vi "py_accel.vi"(7 "Time Target (s)":dbl=1.0, 8 "error in":errorcluster, 10 "Accel CSV file":path, 11 "COM":refnum<visa-resource-name>) -> (2 "File OK":bool, 3 "Com\nError":bool)   [LabVIEW 2021]
uses:
  <vilib>/Instr/_visa.llb/VISA Flush IO Buffer Mask.ctl
panel:
  out "read buffer":string
  # "acc,ms timer refernce,x_accel,y_accel,z_accel   [m/s^2]"
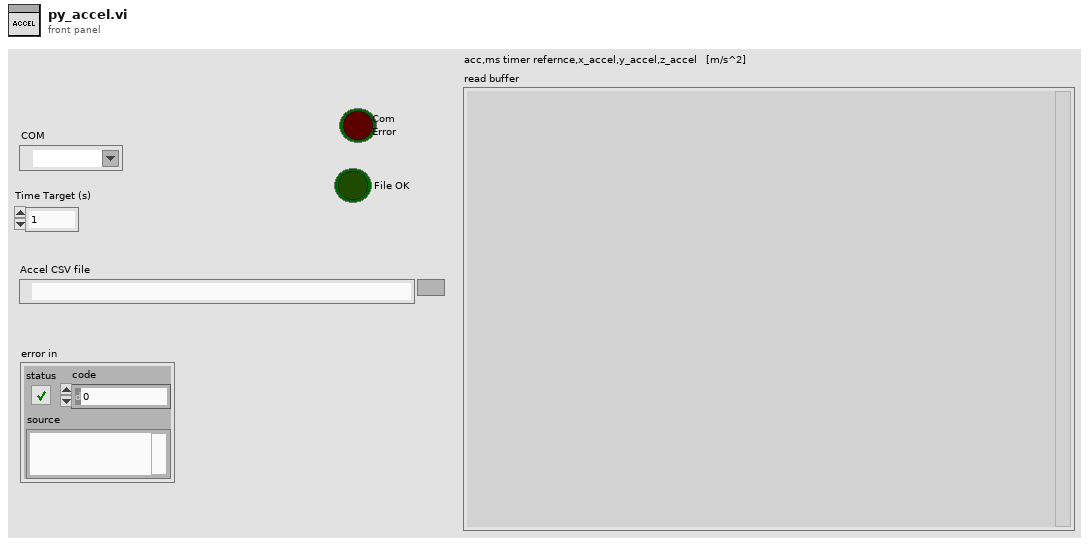
[diagram p1: front panel]
types:
  T1 = typedef "VISA Flush IO Buffer Mask.ctl" = u16
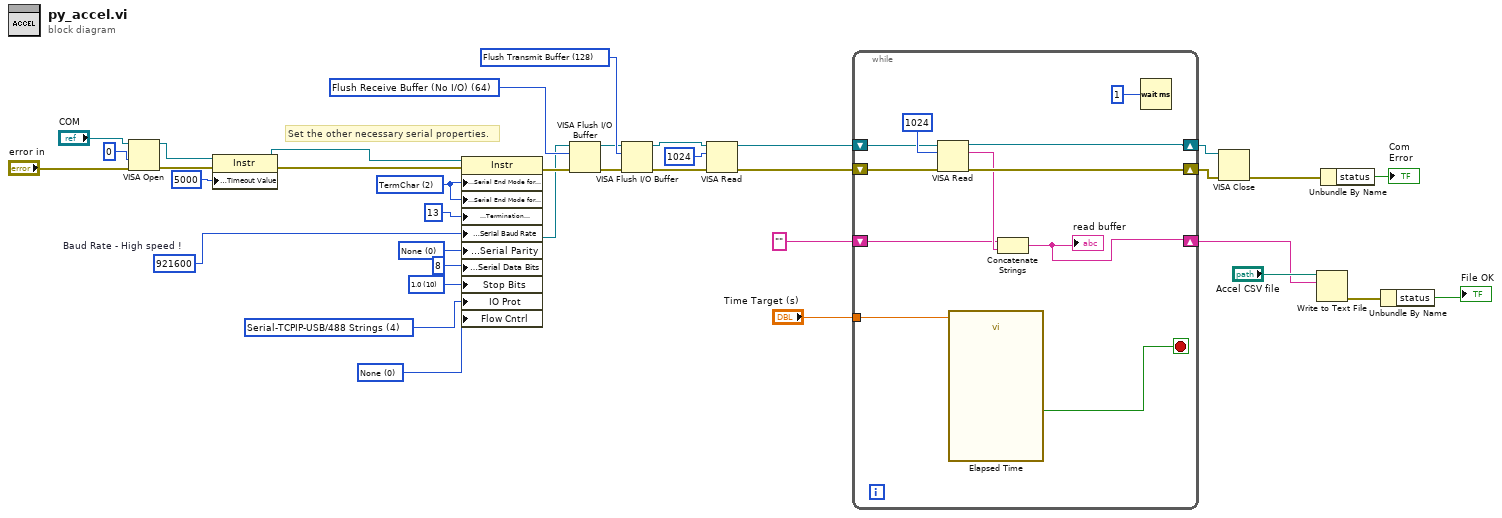
[diagram p0: block diagram]
diagram:
  w11 = u16 0 items=["None", "XON/XOFF", "RTS/CTS", "XON/XOFF & RTS/CTS", "DTR/DSR", "XON/XOFF & DTR/DSR"] ("Serial Settings:Flow Control")
  w12 = u16 0 items=["None", "Odd", "Even", "Mark", "Space"] ("Serial Settings:Parity")
  w14 = u16 10 items=["1.0"=10, "1.5"=15, "2.0"=20] ("Serial Settings:Stop Bits")
  w10 = u32 921600  # Baud Rate - High speed !
  w34 = T1 128 items=["Flush Receive Buffer"=16, "Write Transmit Buffer to Device"=32, "Flush Receive Buffer (No I/O)"=64, "Flush Transmit Buffer"=128] ("Mask")
  w31 = T1 64 items=["Flush Receive Buffer"=16, "Write Transmit Buffer to Device"=32, "Flush Receive Buffer (No I/O)"=64, "Flush Transmit Buffer"=128] ("Mask")
  w26 = u16 2 items=["None", "LastBit", "TermChar"] ("Serial Settings:Serial End Mode for Reads")
  w27 = u16 4 items=["Normal"=1, "VXI/FDC"=2, "GPIB/HS488"=3, "Serial-TCPIP-USB/488 Strings"=4, "USBTMC/Vendor-Specific"=5] ("Message Based Settings:IO Protocol")
  # "Set the other necessary serial properties."
  n1 = VISA Open(access mode=u32 0, error in (no error)="error in", VISA resource name="COM") -> (VISA resource name=w24:refnum<visa-resource-name>, error out=w23:errorcluster)  [unwired: 2 in]
  n2 = property on="Property Node" class="Instr"(reference=w24, error in=w23, "General Settings:Timeout Value"=u32 5000 ("Timeout [ms]")) -> (reference out=w8:refnum<visa-resource-name>, error out=w9:errorcluster)
  n3 = property on="Property Node" class="Instr"(reference=w8, error in=w9, "Serial Settings:Serial End Mode for Reads"=w26, "Serial Settings:Serial End Mode for Writes"=w26, "Message Based Settings:Termination Character"=u8 13, "Serial Settings:Serial Baud Rate"=w10, "Serial Settings:Serial Parity"=w12, "Serial Settings:Serial Data Bits"=u16 8 ("Serial Settings:Data Bits"), "Stop Bits"=w14, "IO Prot"=w27, "Flow Cntrl"=w11) -> (reference out=w29:refnum<visa-resource-name>, error out=w30:errorcluster)
  n4 = VISA Flush I/O Buffer(VISA resource name=w29, mask (16)=w31, error in (no error)=w30) -> (VISA resource name out=w32:refnum<visa-resource-name>, error out=w33:errorcluster)
  n5 = VISA Flush I/O Buffer(VISA resource name=w32, mask (16)=w34, error in (no error)=w33) -> (VISA resource name out=w36:refnum<visa-resource-name>, error out=w37:errorcluster)
  n6 = VISA Read(VISA resource name=w36, byte count=u32 1024, error in (no error)=w37) -> (VISA resource name out=w21:refnum<visa-resource-name>, error out=w20:errorcluster)  [unwired: 2 out]
  n7 = while {
    shift-right: [w45] -> w18
    shift-left: w21 -> [w47]
    shift-right: [w44] -> w17
    shift-left: w20 -> [w46]
    shift-right: [w41] -> w4
    shift-left: "" -> [w42]
    tunnel: "Time Target (s)" -> [w38]
    stop <- w40 stop-if-true
    n8 = VISA Read(VISA resource name=w47, byte count=u32 1024, error in (no error)=w46) -> (VISA resource name out=w45:refnum<visa-resource-name>, read buffer=w43:string, error out=w44:errorcluster)  [unwired: 1 out]
    n9 = call "Elapsed Time"("Time Target (s)"=w38) -> ("Time has Elapsed"=w40:bool)  [unwired: 11 in, 7 out]
    n10 = Concatenate Strings(w42, w43) -> (w41:string)
    "read buffer" <- w41
    n11 = Wait (ms)(milliseconds to wait=u32 1) -> ()  [unwired: 1 out]
  }
  n12 = VISA Close(VISA resource name=w18, error in (no error)=w17) -> (error out=w7:errorcluster)
  n13 = Write to Text File(file (use dialog)="Accel CSV file", text=w4) -> (error out=w3:errorcluster)  [unwired: 2 in, 2 out]
  n14 = Unbundle By Name(w7) -> ("status"=→"Com\nError":bool)
  n15 = Unbundle By Name(w3) -> ("status"=→"File OK":bool)
